vi "Do Core.vi"(8 "error in (no error)":errorcluster, 9 "Actor in":refnum<class "Actor.lvclass">, 11 "Reply Message":refnum<class "Get Bounds and Position Msg.lvclass">) -> (0 "error out":errorcluster, 1 "Actor out":refnum<class "Actor.lvclass">, 2 "Reply":variant)   [LabVIEW 2014, in "ViewableActor.lvlib" / "Get Bounds and Position Msg.lvclass"]
doc: "(<B>Filename</B>: Actor Framework.lvlib:Reply Msg.lvclass:Do Core.vi)\n\nDefines what an actor does when it receives <B>Reply Message</B>. This method also defines the <B>Reply</B> that is returned to the actor that sent <B>Reply Message</B>.\n\nBy default, this method does nothing, and <B>Reply</B> is the ancestor Message class. A child class must override this method to define behavior and specify a child of the Message class to return in the <B>Reply</B> output."
uses:
  Get Bounds and Position Msg.lvclass
  <vilib>/ActorFramework/Actor/Actor.lvclass
  ViewableActor/ViewableActor.lvclass
  ViewableActor/ViewableActor.lvclass/ViewableActor.ctl
  ViewableActor/Read Actor Name.vi
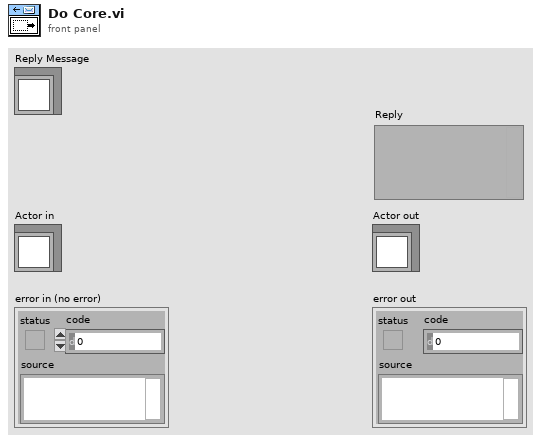
[diagram p1: front panel]
types:
  T1 = typedef "LVRectTypeDef.ctl" = cluster{"Left":i16, "Top":i16, "Right":i16, "Bottom":i16}
  T2 = typedef "LVBoundsTypeDef.ctl" = cluster{"Width":u32, "Height":u32}
  T3 = typedef "LVPositionTypeDef.ctl" = cluster{"Left":i32, "Top":i32}
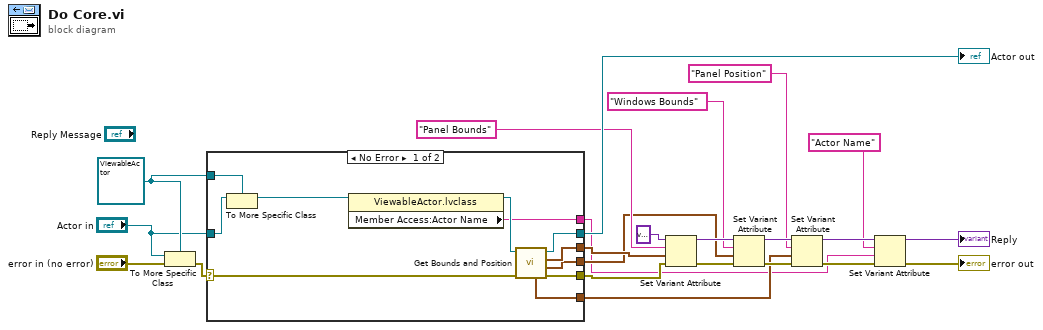
[diagram p0: block diagram]
diagram:
  w23 = refnum<class "ViewableActor.lvclass"> refnum ("Actor in")
  n1 = To More Specific Class(target class=w23, reference="Actor in", error in="error in (no error)") -> (error out=w22:errorcluster)  [unwired: 1 out]
  n2 = case shown="No Error" w22 {
    selector: w22 -> [w32 w36]
    tunnel: [w34 w36] -> w6
    tunnel: [w33 w35] -> w19
    tunnel: "Actor in" -> [w31 w35]
    tunnel: w23 -> [w30 _]
    tunnel: [w28 _] -> w17
    tunnel: [w27 _] -> w12
    tunnel: [w26 _] -> w8
    tunnel: [w24 _] -> w2
    frame No Error {
      n3 = To More Specific Class(target class=w30, reference=w31) -> (specific class reference=w29:refnum<class "ViewableActor.lvclass">)  [unwired: 1 in, 1 out]
      n4 = property class="ViewableActor.lvclass"(reference=w29) -> (reference out=w25:refnum<class "ViewableActor.lvclass">, "Member Access:Actor Name"=w24:string)  [unwired: 1 in, 1 out]
      n5 = call-dynamic "Get Bounds and Position.vi"("error in (no error)"=w32, "ViewableActor in"=w25) -> ("error out"=w34:errorcluster, "Windows Bounds"=w27:T1, "Panel Bounds"=w28:T2, "ViewableActor out"=w33:refnum<class "ViewableActor.lvclass">, "Panel Position"=w26:T3)  [unwired: 5 in]
    }
    frame Error {
      # "If type check fails, pass the original object out again."
    }
  }
  "Actor out" <- w19
  n6 = Set Variant Attribute(Variant=variant ("variant"), name="Panel Bounds", value=w17, error in=w6) -> (Variant out=w18:variant, error out=w9:errorcluster)  [unwired: 1 out]
  n7 = Set Variant Attribute(Variant=w18, name="Windows Bounds", value=w12, error in=w9) -> (Variant out=w14:variant, error out=w10:errorcluster)  [unwired: 1 out]
  n8 = Set Variant Attribute(Variant=w14, name="Panel Position", value=w8, error in=w10) -> (Variant out=w13:variant, error out=w4:errorcluster)  [unwired: 1 out]
  n9 = Set Variant Attribute(Variant=w13, name="Actor Name", value=w2, error in=w4) -> (Variant out=→"Reply":variant, error out=→"error out":errorcluster)  [unwired: 1 out]
